vi "globals.vi"() -> ()   [LabVIEW 2013]
panel:
  in  "Initial phase (degrees)":dbl[](array[numeric])=[0.0, 0.0, 0.0, 0.0, 0.0, 0.0] format="%^#_6g"
  in  "Gain calibration":sgl[][](array[numeric])=[[1.0, 1.0, 1.0, 1.0, 1.0, 1.0], [1.0, 1.0, 1.0, 1.0, 1.0, 1.0], [1.0, 1.0, 1.0, 1.0, 1.0, 1.0], [1.0, 1.0, 1.0, 1.0, 1.0, 1.0], [1.0, 1.0, 1.0, 1.0, 1.0, 1.0], [1.0, 1.0, 1.0, 1.0, 1.0, 1.0], [1.0, 1.0, 1.0, 1.0, 1.0, 1.0], [1.0, 1.0, 1.0, 1.0, 1.0, 1.0]] format="%6.4f"
  in  "Hardware version":T1(ring)=enum."ASAP/Micron 2"
  in  "Phase compensation (degrees)":dbl[][](array[numeric])=[[34.048445792588176, 34.990419035113185, 35.207147246328226, 27.533133442259306], [33.93604501277388, 34.85423748950164, 35.186547618597785, 27.46721375740786], [34.08572539463338, 35.16179529035856, 35.494652560529765, 27.552431969883], [34.044384217116665, 34.987161460355004, 35.57968103290686, 28.088684182699936], [33.86636403387953, 34.97016258659187, 35.414426226767574, 27.79699785215254], [34.02845232993093, 35.2388838636684, 35.75857191246213, 28.15633166530432], [34.07112725184032, 35.31630048013255, 35.77925334149822, 28.014731955001928], [34.21213651524913, 35.355243911895634, 35.96522962202685, 28.565220024397625]] format="%#.1f"
  in  "Phase lags (degrees)":dbl[](array[numeric])=[254.0, 273.5, 326.0, 353.0] format="%^#_6g"
  in  "Num ASAP channels":i32=8
  in  "Repeat interval (samples)":i32=31
  in  "Half periods (sec)":dbl[](array[numeric])=[6.2e-05, 4.96e-05, 3.1e-05, 2.48e-05] format="%#_6p"
  in  "Sample interval (sec)":dbl=1.6e-05 format="%#_6p"
  # "Hardware versions:\nASAP/Trigger: small black-box two-light ASAP w/ trigger output\nASAP/Finder: two-light one-card ASAP config w/finder output, used for calibration under windows\nASAP/Micron: Serial number 1\nASAP/Micron 2: Serial numbers 2,3  Aux digital I/O on the DEV2 port, HV relay\nMicron 6DOF: Serial number 1, with mods.  FPGA LED and motor interface.\n\nAfter modifying these parameters, save them by using testing/save_asap_params.vi.  This creates the asap_params.xml file used by load_asap_params."
  # "Channels"
  # "Frequencies"
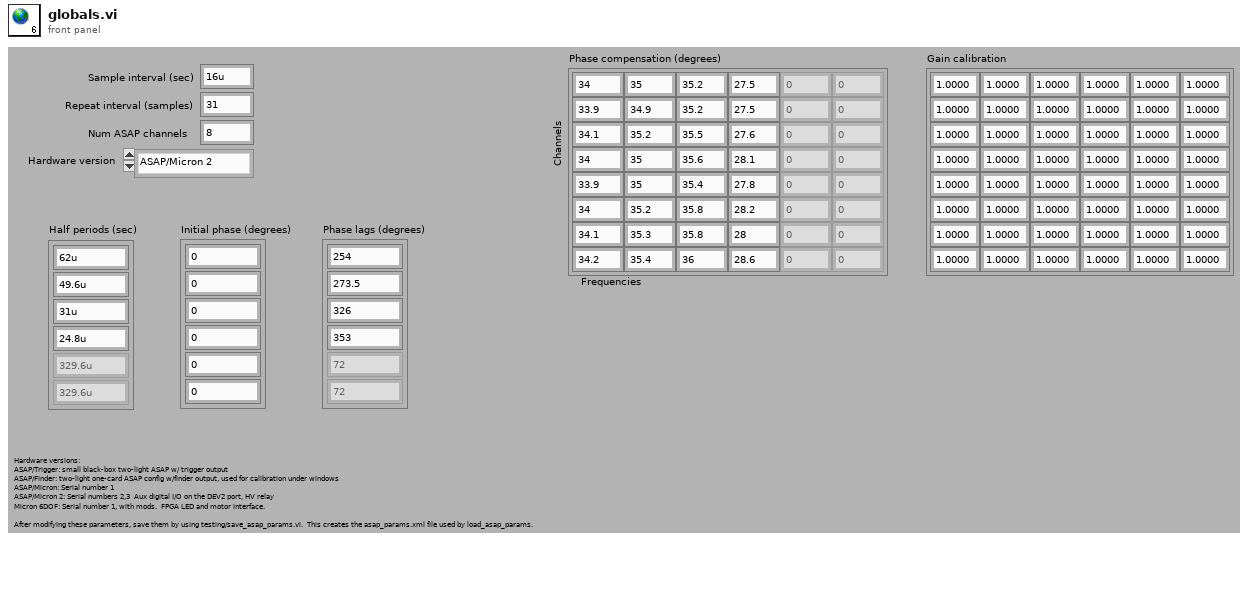
[diagram p1: front panel]
types:
  T1 = enum16{"ASAP/Trigger", "ASAP/Finder", "ASAP/Micron", "ASAP/Micron 2", "Micron 6DOF"}
diagram:
